vi "Wait.vi"(8 "error in (no error)":errorcluster, 9 "Timeout (-1ms)":i32=-1, 11 "Response Msg in":refnum<class "Response Msg.lvclass">) -> (0 "error out":errorcluster, 1 "Timeout?":bool, 3 "Response Msg out":refnum<class "Response Msg.lvclass">)   [LabVIEW 2020, in "Publisher.lvlib" / "Response Msg.lvclass"]
doc: "Execute a Wait using the Wait method of the Response Core."
uses:
  Response Msg.lvclass
  Response Msg.lvclass/Response Msg.ctl
  Response Core/Response Core/Response Core.lvclass
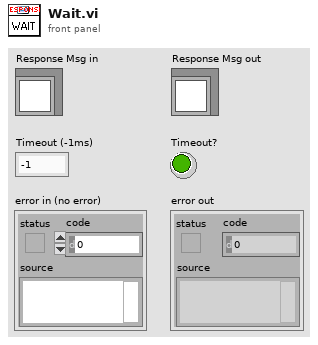
[diagram p1: front panel]
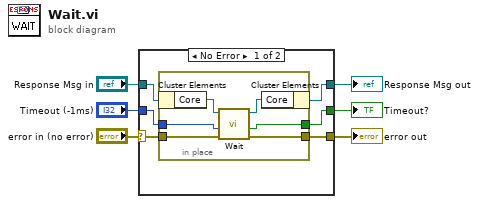
[diagram p0: block diagram]
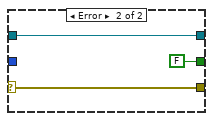
[diagram p2: hidden frame]
diagram:
  n1 = case shown="No Error" "error in (no error)" {
    selector: "error in (no error)" -> [w8 w21]
    tunnel: "Response Msg in" -> [w12 w19]
    tunnel: [w11 w19] -> w5
    tunnel: "Timeout (-1ms)" -> [w10 _]
    tunnel: [w7 w21] -> w2
    tunnel: [w9 FALSE ("Timeout?")] -> w1
    frame No Error {
      n2 = in-place {
        in-place-border: w10 -> [w16]
        in-place-border: [w15] -> w9
        in-place-border: w8 -> [w14]
        in-place-border: [w13] -> w7
        n3 = in-place-cluster #1(w12) -> ("Core"=w18:refnum<class "Response Core.lvclass">)
        n4 = call-dynamic "Wait.vi"("error in (no error)"=w14, "Timeout (-1ms)"=w16, "Response Core in"=w18) -> ("error out"=w13:errorcluster, "Timeout?"=w15:bool, "Response Core out"=w17:refnum<class "Response Core.lvclass">)  [unwired: 6 in]
        n5 = in-place-cluster #1("Core"=w17) -> (w11:refnum<class "Response Msg.lvclass">)
      }
    }
    frame Error {
    }
  }
  "error out" <- w2
  "Response Msg out" <- w5
  "Timeout?" <- w1
